vi "Result_Test.vi"(8 "error in (no error)":errorcluster caption="entrée d'erreur (pas d'erreur)", 11 "Get_Voltage en entrée":refnum<class "Get_SN_DB_AIS.lvclass">) -> (0 "error out":errorcluster caption="sortie d'erreur", 3 "Get_Voltage en sortie":refnum<class "Get_SN_DB_AIS.lvclass">)   [LabVIEW 2020, in "Library Test.lvlib" / "Get_SN_DB_AIS.lvclass"]
uses:
  Get_SN_DB_AIS.lvclass
  C:/Users/ngarcin/OneDrive - Altyor/Standard TB/Class/Test/Test (Default)/Test (Default).lvclass
  Test_Wtih_Instr/Test_With_Inst.lvclass
  Get_SN_DB_AIS.lvclass/Get_SN_DB_AIS.ctl
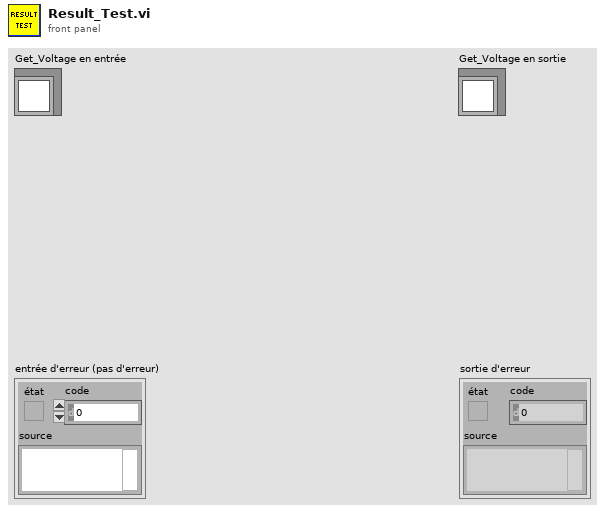
[diagram p1: front panel]
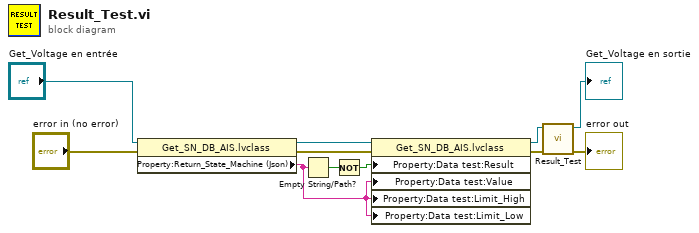
[diagram p0: block diagram]
diagram:
  n1 = property class="Get_SN_DB_AIS.lvclass"(reference="Get_Voltage en entrée", error in="error in (no error)") -> (reference out=w8:refnum<class "Get_SN_DB_AIS.lvclass">, error out=w1:errorcluster, "Property:Return_State_Machine (Json)"=w4:string)
  n2 = Empty String/Path?(string/path=w4) -> (empty?=w3:bool)
  n3 = Not(x=w3) -> (.not. x?=w2:bool)
  n4 = property class="Get_SN_DB_AIS.lvclass"(reference=w8, error in=w1, "Property:Data test:Result"=w2, "Property:Data test:Value"=w4, "Property:Data test:Limit_High"=w4, "Property:Data test:Limit_Low"=w4) -> (reference out=w5:refnum<class "Get_SN_DB_AIS.lvclass">, error out=w6:errorcluster)
  n5 = call-parent "Result_Test.vi"("error in (no error)"=w6, "Test_With_Inst en entrée"=w5) -> ("error out"=→"error out":errorcluster, "Test_With_Inst en sortie"=→"Get_Voltage en sortie":refnum<class "Get_SN_DB_AIS.lvclass">)  [unwired: 8 in]
